vi "Stop.vi"(8 "Error In":errorcluster, 11 "object in":refnum<class "Teledyne-T3AFG120.lvclass">=refnum) -> (0 "Error Out":errorcluster, 3 "object out":refnum<class "Teledyne-T3AFG120.lvclass">)   [LabVIEW 2023, in "Teledyne-T3AFG120.lvlib" / "Teledyne-T3AFG120.lvclass"]
uses:
  Teledyne-T3AFG120.lvclass
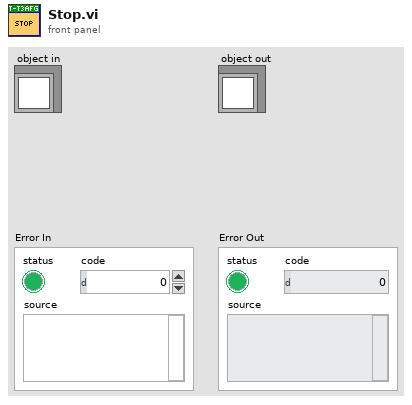
[diagram p1: front panel]
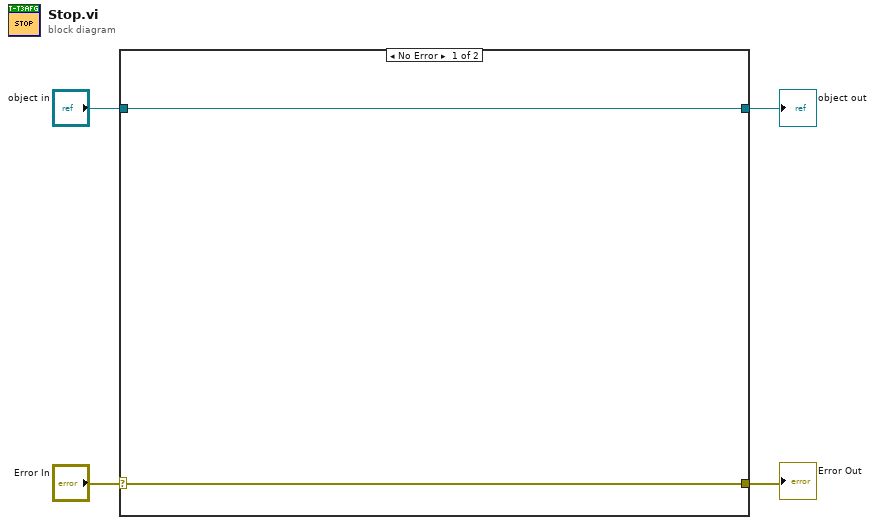
[diagram p0: block diagram]
diagram:
  n1 = case shown="No Error" "Error In" {
    selector: "Error In" -> [w6 w8]
    tunnel: [w6 w8] -> w3
    tunnel: [w5 w7] -> w1
    tunnel: "object in" -> [w5 w7]
    frame No Error {
    }
    frame Error {
    }
  }
  "Error Out" <- w3
  "object out" <- w1
